vi "GPS Type.vi"(11 "Nema Def":string) -> (2 "RTK = T":bool, 3 "GPS Type":string)   [LabVIEW 2012]
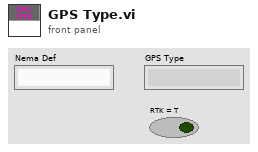
[diagram p1: front panel]
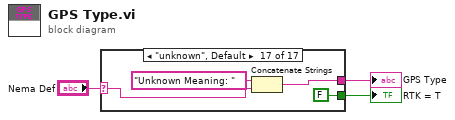
[diagram p0: block diagram]
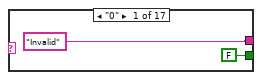
[diagram p2: hidden frame]
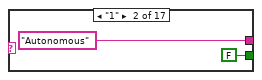
[diagram p3: hidden frame]
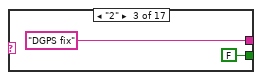
[diagram p4: hidden frame]
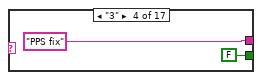
[diagram p5: hidden frame]
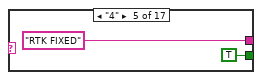
[diagram p6: hidden frame]
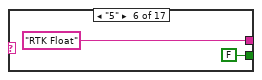
[diagram p7: hidden frame]
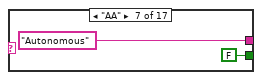
[diagram p8: hidden frame]
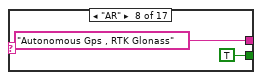
[diagram p9: hidden frame]
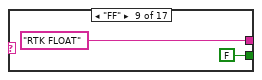
[diagram p10: hidden frame]
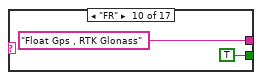
[diagram p11: hidden frame]
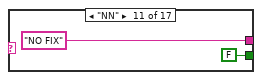
[diagram p12: hidden frame]
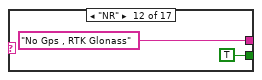
[diagram p13: hidden frame]
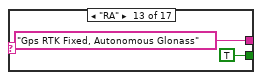
[diagram p14: hidden frame]
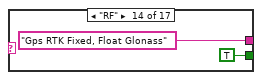
[diagram p15: hidden frame]
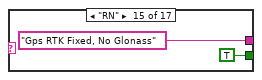
[diagram p16: hidden frame]
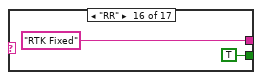
[diagram p17: hidden frame]
diagram:
  n1 = case shown="\"unknown\", Default" "Nema Def" {
    selector: "Nema Def" -> [_ _ _ _ _ _ _ _ _ _ _ _ _ _ _ _ w37]
    tunnel: ["Invalid" "Autonomous" "DGPS fix" "PPS fix" "RTK FIXED" "RTK Float" "Autonomous" "Autonomous Gps , RTK Glonass" "RTK FLOAT" "Float Gps , RTK Glonass" "NO FIX" "No Gps , RTK Glonass" "Gps RTK Fixed, Autonomous Glonass" "Gps RTK Fixed, Float Glonass" "Gps RTK Fixed, No Glonass" "RTK Fixed" w38] -> w3
    tunnel: [FALSE FALSE FALSE FALSE TRUE FALSE FALSE TRUE FALSE TRUE FALSE TRUE TRUE TRUE TRUE TRUE FALSE] -> w2
    frame "0" {
    }
    frame "1" {
    }
    frame "2" {
    }
    frame "3" {
    }
    frame "4" {
    }
    frame "5" {
    }
    frame "AA" {
    }
    frame "AR" {
    }
    frame "FF" {
    }
    frame "FR" {
    }
    frame "NN" {
    }
    frame "NR" {
    }
    frame "RA" {
    }
    frame "RF" {
    }
    frame "RN" {
    }
    frame "RR" {
    }
    frame "unknown", Default {
      n2 = Concatenate Strings("Unknown Meaning: ", w37) -> (w38:string)
    }
  }
  "GPS Type" <- w3
  "RTK = T" <- w2
